vi "Compute Max Level.vi"(0 "Noise in":refnum<class "Noise.lvclass">, 1 "Filter in":refnum<class "Filter.lvclass">, 5 "Level in":refnum<class "Level.lvclass">, 7 "Fs (Hz)":dbl, 9 "Vmax":dbl, 11 "error in (no error)":errorcluster) -> (4 "Noise out":refnum<class "Noise.lvclass">, 6 "Level thru":refnum<class "Level.lvclass">, 10 "Lmax":dbl, 15 "error out":errorcluster)   [LabVIEW 2020, in "Noise.lvclass"]
uses:
  Noise.lvclass
  D:/Development/epl-vi-lib/Koop/KObject Class/KObject.lvclass
  Level/Level.lvclass
  Filter/Filter.lvclass
  Level/LevelUnits.ctl
  Noise.lvclass/Noise.ctl
  Level/Level.lvclass/Level.ctl
  <vilib>/Analysis/5stat.llb/RMS (DBL).vi
  6d177499-f940-4193-b657-3015f7a6ed09.vi
  b8aab703-8731-46b6-b9eb-ab2ebcb88006.vi
  5eddbcbb-84d1-4565-8344-307b6f2d13f6.vi
  a2929a10-7a8c-4bed-a29e-c4a8951e9c18.vi
  Filter/Read Class.vi
  Level/Read Units.vi
  Koop/KObject Class/KObject.lvclass
  <vilib>/Analysis/NI_AALPro.lvlib
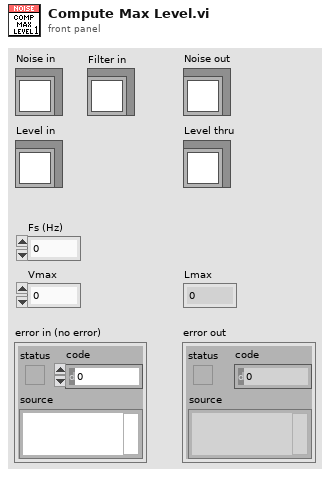
[diagram p1: front panel]
types:
  T1 = typedef "Level.lvclass/LevelUnits.ctl" = enum16{"dB atten", "dB SPL", "dB Vrms", "Volts", "dB mW", "mW", "dB HL", "dB SL"}
  T2 = enum16{"Clear", "Set data", "Reset index", "Get data"}
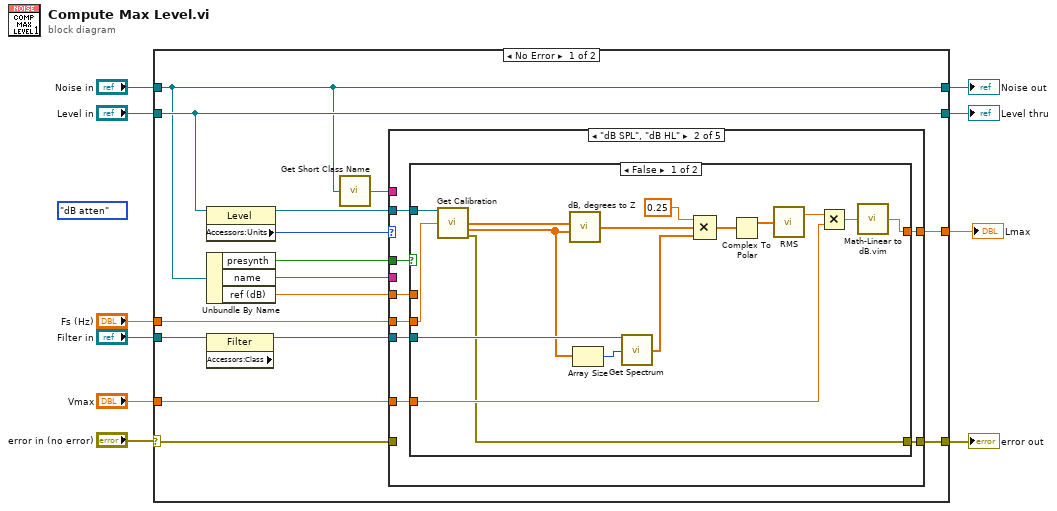
[diagram p0: block diagram]
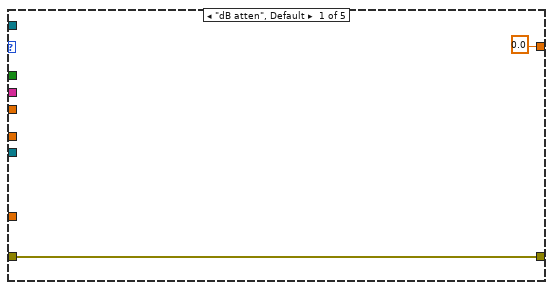
[diagram p2: hidden frame]
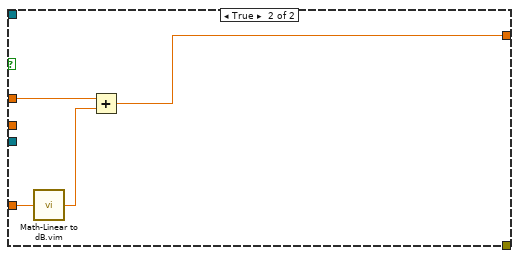
[diagram p3: hidden frame]
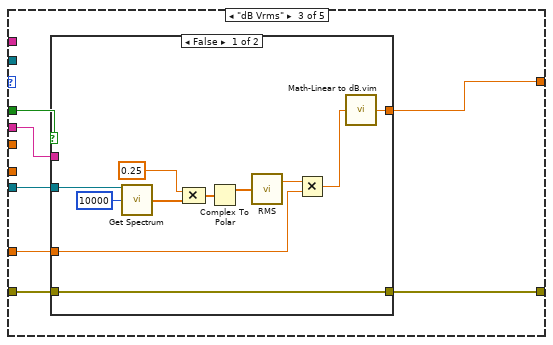
[diagram p4: hidden frame]
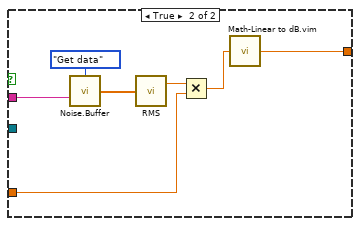
[diagram p5: hidden frame]
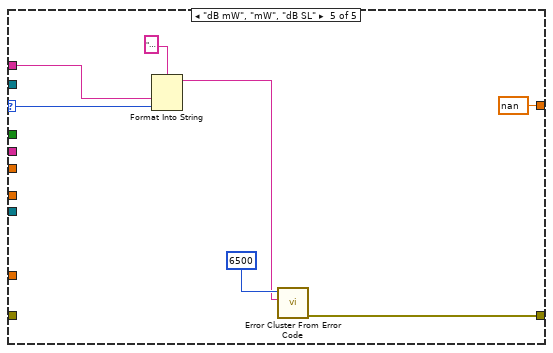
[diagram p7: hidden frame]
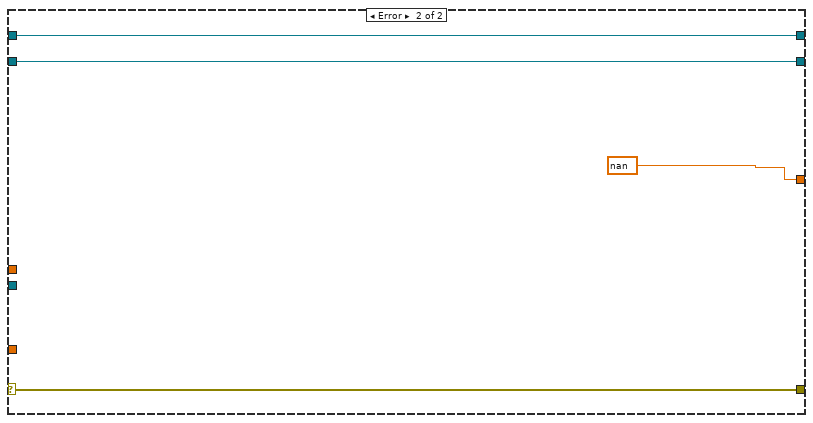
[diagram p8: hidden frame]
diagram:
  (unwired) LevelUnits."dB atten" ("Units")
  n1 = case shown="No Error" "error in (no error)" {
    selector: "error in (no error)" -> [w16 w91]
    tunnel: [w18 w93] -> w5
    tunnel: "Noise in" -> [w18 w93]
    tunnel: [w25 w92] -> w6
    tunnel: "Level in" -> [w25 w92]
    tunnel: "Vmax" -> [w20 _]
    tunnel: [w19 w91] -> w4
    tunnel: [w21 nan] -> w7
    tunnel: "Filter in" -> [w14 _]
    tunnel: "Fs (Hz)" -> [w12 _]
    frame No Error {
      n2 = property class="Level"(reference=w25) -> (reference out=w22:refnum<class "Level.lvclass">, "Accessors:Units"=w24:T1)  [unwired: 1 in, 1 out]
      n3 = Unbundle By Name(w18) -> ("presynth"=w15:bool, "name"=w23:string, "ref (dB)"=w11:dbl)
      n4 = property class="Filter" props=["Accessors:Class"](reference=w14) -> (reference out=w13:refnum<class "Filter.lvclass">)  [unwired: 1 in, 2 out]
      n5 = call "Get Short Class Name.vi"("KObject in"=w18) -> ("Class"=w17:string)  [unwired: 4 in]
      n6 = case shown="\"dB SPL\", \"dB HL\"" w24 {
        selector: w24 -> [_ _ _ _ w84]
        tunnel: w23 -> [_ _ w56 _ _]
        tunnel: w22 -> [_ w32 _ _ _]
        tunnel: [0.0 w33 w61 w82 nan ("Vmax")] -> w21
        tunnel: w20 -> [_ w34 w62 w82 _]
        tunnel: [w26 w31 w58 w81 w85] -> w19
        tunnel: w17 -> [_ _ _ _ w83]
        tunnel: w16 -> [w26 _ w59 w81 _]
        tunnel: w15 -> [_ w29 w60 _ _]
        tunnel: w13 -> [_ w35 w57 _ _]
        tunnel: w12 -> [_ w30 _ _ _]
        tunnel: w11 -> [_ w28 _ _ _]
        frame "dB atten", Default {
        }
        frame "dB SPL", "dB HL" {
          n7 = case shown="False" w29 {
            tunnel: w35 -> [w47 _]
            tunnel: w34 -> [w43 w55]
            tunnel: [w42 w52] -> w33
            tunnel: w32 -> [w40 _]
            tunnel: [w39 _] -> w31
            tunnel: w30 -> [w38 _]
            tunnel: w28 -> [_ w54]
            frame False {
              n8 = call "Get Calibration.vi"("Level in"=w40, "Fs (Hz)"=w38) -> ("Mag (dB SPL)"=w37:dbl[], "Phase (degrees)"=w36:dbl[], "error out"=w39:errorcluster)  [unwired: 9 in, 2 out]
              n9 = call "dB, degrees to Z.vi"("Magnitude (dB)"=w37, "Phase (degrees)"=w36) -> ("Z"=w46:cdb[])  [unwired: 5 in]
              n10 = Array Size(array=w36) -> (size(s)=w48:i32)
              n11 = call "Get Spectrum.vi"("Filter in"=w47, "Npts"=w48) -> ("spectrum"=w41:cdb[])  [unwired: 11 in, 2 out]
              n12 = Compound Arithmetic op=MULTIPLY(0.25, w46, w41) -> (w44:cdb[])
              n13 = Complex To Polar(r * e^(i*theta)=w44) -> (r=w51:dbl[])  [unwired: 1 out]
              n14 = call-poly <vilib>:"RMS.vi"("X"=w51) -> ("rms value"=w50:dbl)  [unwired: 1 out]
              n15 = Multiply(x=w50, y=w43) -> (x*y=w49:dbl)
              n16 = call "Math-Linear to dB.vim"("linear"=w49) -> ("dB"=w42:dbl)
            }
            frame True {
              n17 = call "Math-Linear to dB.vim"("linear"=w55) -> ("dB"=w53:dbl)
              n18 = Add(x=w54, y=w53) -> (x+y=w52:dbl)
            }
          }
        }
        frame "dB Vrms" {
          n19 = case shown="False" w60 {
            tunnel: w62 -> [w65 w75]
            tunnel: [w73 w74] -> w61
            tunnel: w59 -> [w72 _]
            tunnel: [w72 _] -> w58
            tunnel: w57 -> [w71 _]
            tunnel: w56 -> [_ w79]
            frame False {
              n20 = call "Get Spectrum.vi"("Filter in"=w71, "Npts"=10000) -> ("spectrum"=w68:cdb[])  [unwired: 11 in, 2 out]
              n21 = Compound Arithmetic op=MULTIPLY(0.25, w68) -> (w69:cdb[])
              n22 = Complex To Polar(r * e^(i*theta)=w69) -> (r=w70:dbl[])  [unwired: 1 out]
              n23 = call-poly <vilib>:"RMS.vi"("X"=w70) -> ("rms value"=w66:dbl)  [unwired: 1 out]
              n24 = Multiply(x=w66, y=w65) -> (x*y=w64:dbl)
              n25 = call "Math-Linear to dB.vim"("linear"=w64) -> ("dB"=w73:dbl)
            }
            frame True {
              n26 = call "Noise.Buffer.vi"("Action"=T2."Get data", "Name"=w79) -> ("Data Out"=w76:dbl[])  [unwired: 12 in, 1 out]
              n27 = call-poly <vilib>:"RMS.vi"("X"=w76) -> ("rms value"=w78:dbl)  [unwired: 1 out]
              n28 = Multiply(x=w78, y=w75) -> (x*y=w77:dbl)
              n29 = call "Math-Linear to dB.vim"("linear"=w77) -> ("dB"=w74:dbl)
            }
          }
        }
        frame "Volts" {
        }
        frame "dB mW", "mW", "dB SL" {
          n30 = Format Into String(format string="%s: Cannot set level in '%s'", w83, w84) -> (resulting string=w86:string)  [unwired: 2 in, 1 out]
          n31 = call <vilib>:"Error Cluster From Error Code.vi"("error message (\"\")"=w86, "error code (0)"=6500) -> ("error out"=w85:errorcluster)  [unwired: 7 in]
        }
      }
    }
    frame Error {
    }
  }
  "error out" <- w4
  "Noise out" <- w5
  "Level thru" <- w6
  "Lmax" <- w7
